vi "Coeficientes da norma - Uniforme.vi"(1 "Método de análise":T1(ring)=enum."Simplificado 2008", 2 "Tipo de roseta":u16(ring) items=["Roseta A", "Roseta B", "Roseta C"], 3 "Coluna":dbl=0.45 format="%#_13g", 4 "Linha":dbl=0.05 format="%#_13g") -> (0 "Coeficiente a e b":dbl[](array[numeric]))   [LabVIEW 2016]
uses:
  <vilib>/gmath/NI_Gmath.lvlib
panel:
  out "Linha":dbl[](array[numeric])
  out "Coluna":dbl[](array[numeric])
  out "Coeficiente B":dbl[][](array[numeric])
  out "Coeficiente A":dbl[][](array[numeric])
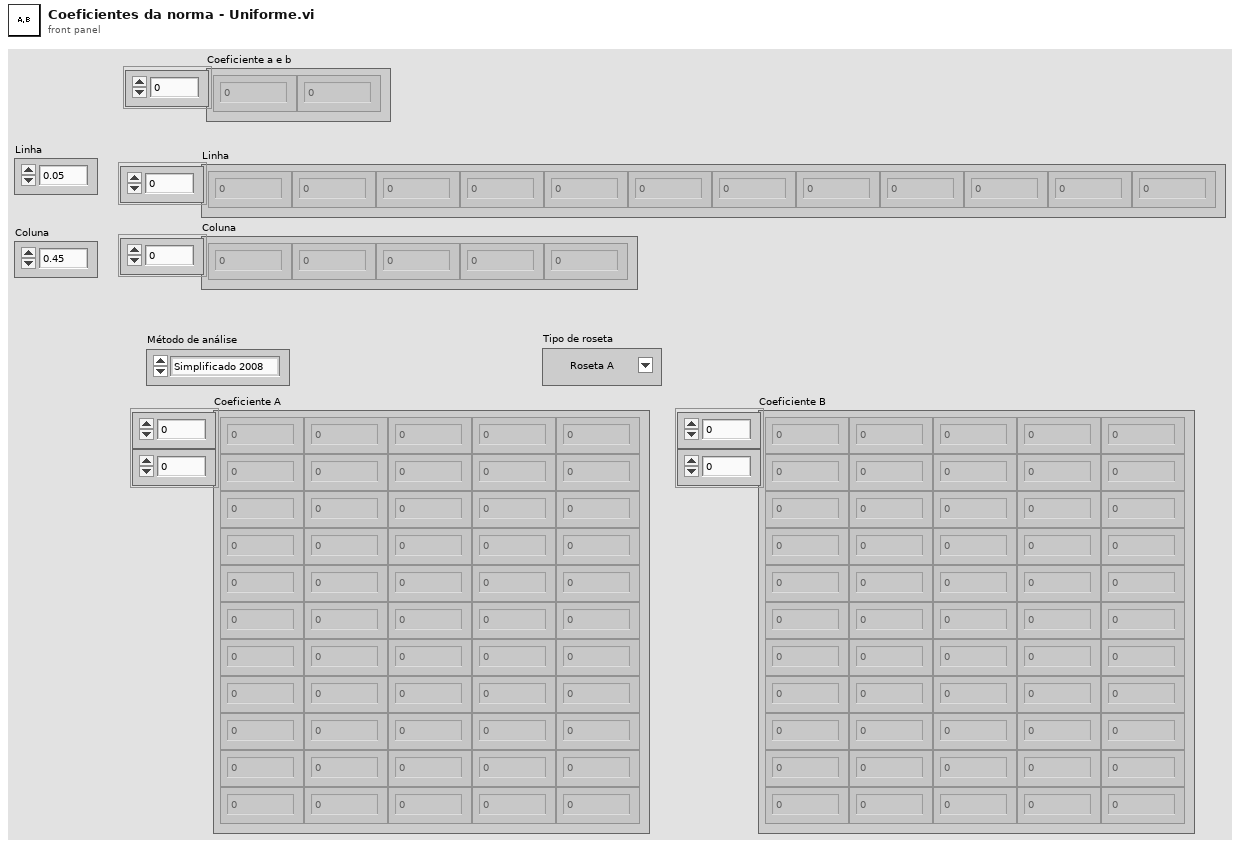
[diagram p1: front panel]
types:
  T1 = enum16{"Não uniforme 2013", "Simplificado 2013", "Simplificado 2008"}
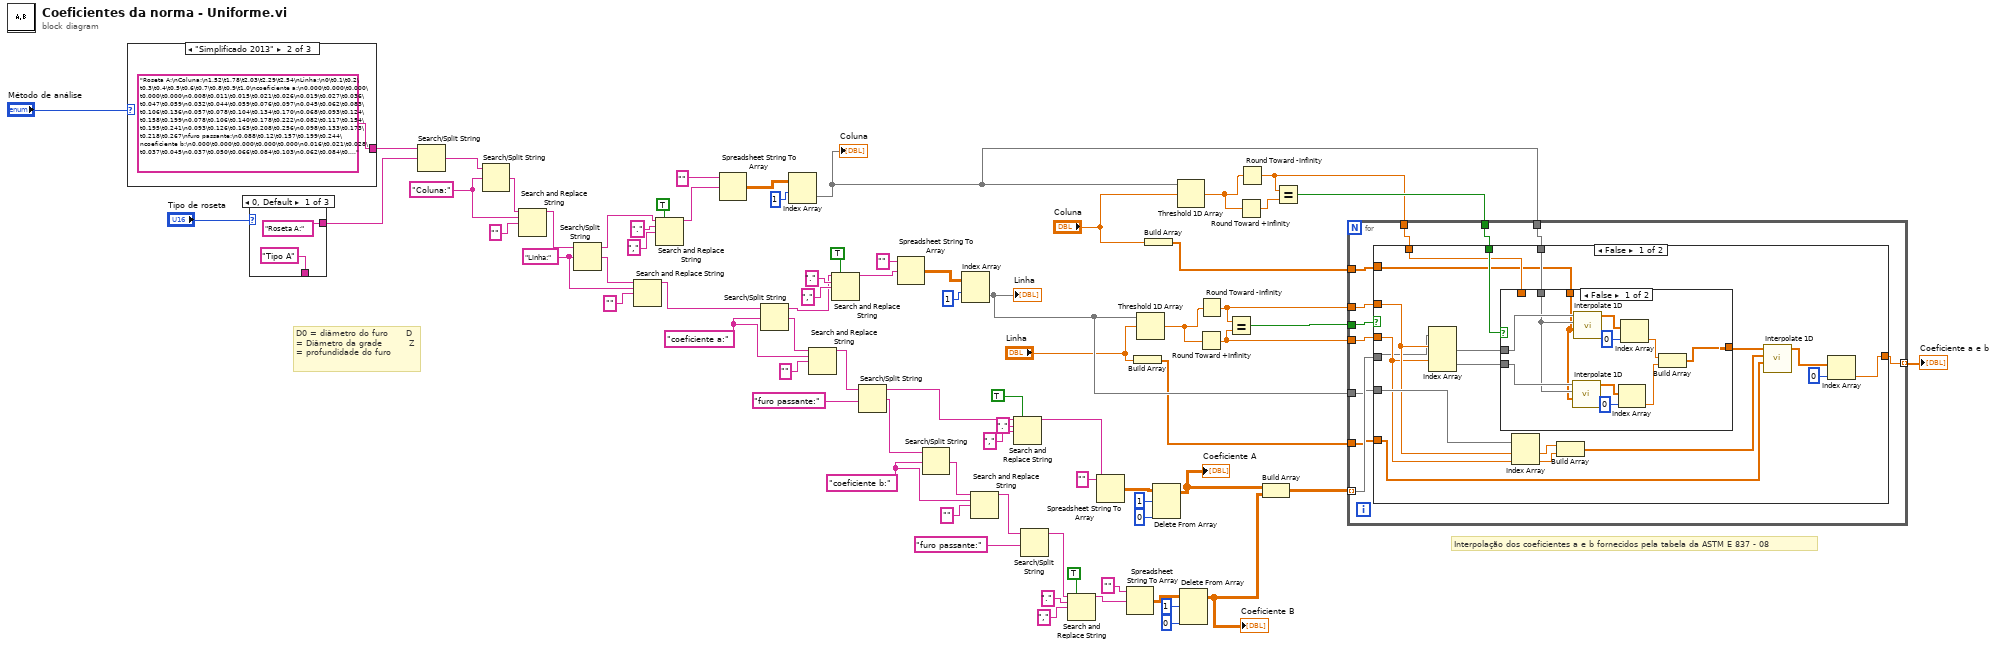
[diagram p0: block diagram]
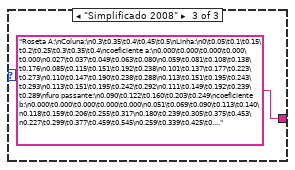
[diagram p3: hidden frame]
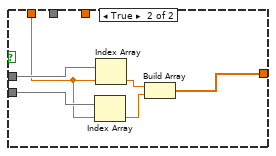
[diagram p4: hidden frame]
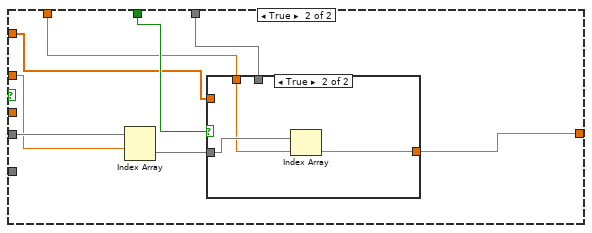
[diagram p5: hidden frame]
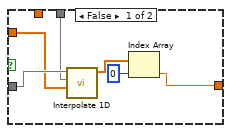
[diagram p6: hidden frame]
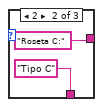
[diagram p7: hidden frame]
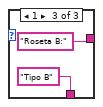
[diagram p8: hidden frame]
diagram:
  w40 = "Linha:" ("search string/char (-)")
  w42 = "Coluna:" ("search string/char (-)")
  w65 = "coeficiente b:"
  w74 = "coeficiente a:"
  # "Interpolação dos coeficientes a e b fornecidos pela tabela da ASTM E 837 - 08"
  # "D0 = diâmetro do furo      D = Diâmetro da grade         Z = profundidade do furo"
  n1 = case shown="\"Simplificado 2013\"" "Método de análise" {
    tunnel: [_ "Roseta A:\nColuna:\n1.52\t1.78\t2.03\t2.29\t2.54\nLinha:\n0\t0.1\t0.2\t0.3\t0.4\t0.5\t0.6\t0.7\t0.8\t0.9\t1.0\ncoeficiente a:\n0.000\t0.000\t0.000\t0.000\t0.000\n0.008\t0.011\t0.015\t0.021\t0.026\n0.019\t0.027\t0.036\t0.047\t0.059\n0.032\t0.044\t0.059\t0.076\t0.097\n0.045\t0.062\t0.083\t0.106\t0.136\n0.057\t0.078\t0.104\t0.134\t0.170\n0.068\t0.093\t0.124\t0.158\t0.199\n0.078\t0.106\t0.140\t0.178\t0.222\n0.082\t0.117\t0.154\t0.195\t0.241\n0.093\t0.126\t0.165\t0.208\t0.256\n0.098\t0.133\t0.173\t0.218\t0.267\nfuro passante:\n0.088\t0.12\t0.157\t0.199\t0.244\ncoeficiente b:\n0.000\t0.000\t0.000\t0.000\t0.000\n0.016\t0.021\t0.028\t0.037\t0.045\n0.037\t0.050\t0.066\t0.084\t0.103\n0.062\t0.084\t0.110\t0.137\t0.171\n0.088\t0.119\t0.155\t0.193\t0.241\n0.115\t0.154\t0.200\t0.248\t0.307\n0.140\t0.187\t0.242\t0.299\t0.367\n0.164\t0.218\t0.280\t0.345\t0.418\n0.185\t0.246\t0.314\t0.385\t0.463\n0.204\t0.270\t0.343\t0.419\t0.501\n0.221\t0.291\t0.370\t0.449\t0.533\nfuro passante:\n0.283\t0.371\t0.463\t0.554\t0.642\nCurvas limites:\ninferior:\n0\t0.1851\t0.4283\t0.6319\t0.7804\t0.8812\t0.9405\t0.9786\t1\nsuperior:\n0\t0.2559\t0.5602\t0.7845\t0.9198\t0.9874\t10.0143\t10.0143\t1 \n;\nRoseta B:\nColuna:\n1.52\t1.78\t2.03\t2.29\t2.54\nLinha:\n0\t0.1\t0.2\t0.3\t0.4\t0.5\t0.6\t0.7\t0.8\t0.9\t1.0\ncoeficiente a:\n0.000\t0.000\t0.000\t0.000\t0.000\n0.009\t0.012\t0.016\t0.022\t0.027\n0.021\t0.029\t0.039\t0.051\t0.063\n0.034\t0.047\t0.064\t0.082\t0.105\n0.048\t0.066\t0.089\t0.114\t0.146\n0.061\t0.084\t0.112\t0.143\t0.183\n0.073\t0.100\t0.132\t0.169\t0.213\n0.083\t0.114\t0.150\t0.190\t0.237\n0.092\t0.125\t0.164\t0.207\t0.256\n0.099\t0.134\t0.175\t0.221\t0.271\n0.105\t0.142\t0.184\t0.231\t0.282\nfuro passante:\n0.094\t0.128\t0.167\t0.212\t0.260\ncoeficiente b:\n0.000\t0.000\t0.000\t0.000\t0.000\n0.018\t0.024\t0.032\t0.041\t0.050\n0.042\t0.057\t0.074\t0.093\t0.115\n0.070\t0.094\t0.123\t0.153\t0.191\n0.100\t0.134\t0.175\t0.216\t0.270\n0.130\t0.174\t0.225\t0.278\t0.343\n0.159\t0.211\t0.272\t0.335\t0.409\n0.185\t0.246\t0.314\t0.385\t0.466\n0.209\t0.277\t0.352\t0.430\t0.515\n0.231\t0.305\t0.385\t0.468\t0.557\n0.249\t0.328\t0.413\t0.500\t0.592\nfuro passante:\n0.322\t0.421\t0.523\t0.621\t0.716\nCurvas limites:\ninferior:\n0\t0.1878\t0.4255\t0.6349\t0.7818\t0.8809\t0.9430\t0.9785\t1\nsuperior:\n0\t0.2623\t0.5695\t0.7966\t0.9297\t0.9964\t10.0143\t10.0136\t1\n;\nRoseta C:\nColuna:\n1.52\t1.78\t2.03\t2.29\t2.54\nLinha:\n0\t0.1\t0.2\t0.3\t0.4\t0.5\t0.6\t0.7\t0.8\t0.9\t1.0\ncoeficiente a:\n0.000\t0.000\t0.000\t0.000\t0.000\n0.019\t0.027\t0.038\t0.050\t0.061\n0.046\t0.064\t0.086\t0.111\t0.139\n0.076\t0.105\t0.141\t0.182\t0.235\n0.106\t0.147\t0.197\t0.253\t0.324\n0.134\t0.186\t0.248\t0.316\t0.400\n0.160\t0.221\t0.292\t0.371\t0.464\n0.182\t0.250\t0.330\t0.416\t0.515\n0.201\t0.275\t0.361\t0.453\t0.556\n0.217\t0.296\t0.386\t0.482\t0.588\n0.230\t0.312\t0.405\t0.505\t0.613\nfuro passante:\n0.246\t0.335\t0.437\t0.553\t0.681\ncoeficiente b:\n0.000\t0.000\t0.000\t0.000\t0.000\n0.032\t0.043\t0.056\t0.070\t0.082\n0.076\t0.103\t0.132\t0.161\t0.193\n0.128\t0.172\t0.221\t0.269\t0.333\n0.184\t0.246\t0.315\t0.383\t0.468\n0.240\t0.320\t0.407\t0.490\t0.589\n0.293\t0.389\t0.491\t0.587\t0.695\n0.343\t0.452\t0.566\t0.673\t0.784\n0.387\t0.507\t0.631\t0.745\t0.858\n0.427\t0.556\t0.687\t0.806\t0.918\n0.461\t0.597\t0.734\t0.856\t0.968\nfuro passante:\n0.519\t0.648\t0.758\t0.831\t0.860\nCurvas limites:\ninferior:\n0\t0.1632\t0.3793\t0.5860\t0.7365\t0.8482\t0.9213\t0.9680\t1\nsuperior:\n0\t0.2079\t0.4643\t0.6754\t0.8238\t0.9099\t0.9608\t0.9844\t1\n;" ("text") "Roseta A:\nColuna:\n0.3\t0.35\t0.4\t0.45\t0.5\nLinha:\n0\t0.05\t0.1\t0.15\t0.2\t0.25\t0.3\t0.35\t0.4\ncoeficiente a:\n0.000\t0.000\t0.000\t0.000\t0.000\n0.027\t0.037\t0.049\t0.063\t0.080\n0.059\t0.081\t0.108\t0.138\t0.176\n0.085\t0.115\t0.151\t0.192\t0.238\n0.101\t0.137\t0.177\t0.223\t0.273\n0.110\t0.147\t0.190\t0.238\t0.288\n0.113\t0.151\t0.195\t0.243\t0.293\n0.113\t0.151\t0.195\t0.242\t0.292\n0.111\t0.149\t0.192\t0.239\t0.289\nfuro passante:\n0.090\t0.122\t0.160\t0.203\t0.249\ncoeficiente b:\n0.000\t0.000\t0.000\t0.000\t0.000\n0.051\t0.069\t0.090\t0.113\t0.140\n0.118\t0.159\t0.206\t0.255\t0.317\n0.180\t0.239\t0.305\t0.375\t0.453\n0.227\t0.299\t0.377\t0.459\t0.545\n0.259\t0.339\t0.425\t0.513\t0.603\n0.279\t0.364\t0.454\t0.546\t0.638\n0.292\t0.379\t0.472\t0.566\t0.657\n0.297\t0.387\t0.482\t0.576\t0.668\nfuro passante:\n0.288\t0.377\t0.470\t0.562\t0.651\nCurvas limites:\ninferior:\n0\t0.1851\t0.4283\t0.6319\t0.7804\t0.8812\t0.9405\t0.9786\t1\nsuperior:\n0\t0.2559\t0.5602\t0.7845\t0.9198\t0.9874\t10.0143\t10.0143\t1 \n;\nRoseta B:\nColuna:\n0.3\t0.35\t0.4\t0.45\t0.5\nLinha:\n0\t0.05\t0.1\t0.15\t0.2\t0.25\t0.3\t0.35\t0.4\ncoeficiente a:\n0.000\t0.000\t0.000\t0.000\t0.000\n0.029\t0.039\t0.053\t0.068\t0.086\n0.063\t0.087\t0.116\t0.148\t0.189\n0.090\t0.123\t0.162\t0.205\t0.254\n0.107\t0.145\t0.189\t0.236\t0.289\n0.116\t0.156\t0.202\t0.251\t0.305\n0.120\t0.160\t0.206\t0.256\t0.309\n0.120\t0.160\t0.206\t0.256\t0.308\n0.118\t0.158\t0.203\t0.253\t0.305\nfuro passante:\n0.096\t0.131\t0.171\t0.216\t0.265\ncoeficiente b:\n0.000\t0.000\t0.000\t0.000\t0.000\n0.058\t0.078\t0.102\t0.127\t0.157\n0.134\t0.179\t0.231\t0.286\t0.355\n0.203\t0.269\t0.343\t0.419\t0.504\n0.256\t0.336\t0.423\t0.511\t0.605\n0.292\t0.381\t0.476\t0.571\t0.668\n0.315\t0.410\t0.509\t0.609\t0.707\n0.330\t0.427\t0.529\t0.631\t0.730\n0.337\t0.437\t0.541\t0.644\t0.743\nfuro passante:\n0.329\t0.428\t0.531\t0.630\t0.725\nCurvas limites:\ninferior:\n0\t0.1878\t0.4255\t0.6349\t0.7818\t0.8809\t0.9430\t0.9785\t1\nsuperior:\n0\t0.2623\t0.5695\t0.7966\t0.9297\t0.9964\t10.0143\t10.0136\t1\n;\nRoseta C:\nColuna:\n0.4\t0.45\t0.5\t0.55\t0.6\nLinha:\n0\t0.05\t0.1\t0.15\t0.2\t0.25\t0.3\t0.35\t0.4\ncoeficiente a:\n0.000\t0.000\t0.000\t0.000\t0.000\n0.065\t0.084\t0.106\t0.130\t0.157\n0.147\t0.191\t0.238\t0.293\t0.361\n0.218\t0.281\t0.347\t0.420\t0.506\n0.270\t0.343\t0.421\t0.504\t0.595\n0.302\t0.381\t0.465\t0.554\t0.648\n0.321\t0.403\t0.491\t0.583\t0.679\n0.331\t0.415\t0.505\t0.599\t0.698\n0.336\t0.421\t0.512\t0.608\t0.709\nfuro passante:\n0.316\t0.399\t0.494\t0.597\t0.707\ncoeficiente b:\n0.000\t0.000\t0.000\t0.000\t0.000\n0.105\t0.132\t0.158\t0.185\t0.217\n0.250\t0.314\t0.373\t0.440\t0.519\n0.391\t0.484\t0.570\t0.658\t0.754\n0.506\t0.617\t0.719\t0.816\t0.912\n0.591\t0.712\t0.823\t0.923\t10.015\n0.650\t0.778\t0.893\t0.994\t10.081\n0.690\t0.822\t0.939\t10.041\t10.125\n0.719\t0.851\t0.970\t10.073\t10.154\nfuro passante:\n0.623\t0.723\t0.799\t0.847\t0.859\nCurvas limites:\ninferior:\n0\t0.1632\t0.3793\t0.5860\t0.7365\t0.8482\t0.9213\t0.9680\t1\nsuperior:\n0\t0.2079\t0.4643\t0.6754\t0.8238\t0.9099\t0.9608\t0.9844\t1\n;" ("text")] -> w2
    frame "Não uniforme 2013", Default {
    }
    frame "Simplificado 2013" {
    }
    frame "Simplificado 2008" {
    }
  }
  n2 = case shown="0, Default" "Tipo de roseta" {
    tunnel: ["Roseta A:" "Roseta C:" "Roseta B:"] -> w75
    tunnel: ["Tipo A" "Tipo C" "Tipo B"] -> _
    frame 0, Default {
    }
    frame 2 {
    }
    frame 1 {
    }
  }
  n3 = Search/Split String(string=w2, search string/char (-)=w75) -> (match + rest of string=w45:string)  [unwired: 1 in, 2 out]
  n4 = Search/Split String(string=w45, search string/char (-)=w42) -> (match + rest of string=w43:string)  [unwired: 1 in, 2 out]
  n5 = Search and Replace String(input string=w43, search string=w42, replace string="" ("replace string (\"\")")) -> (result string=w38:string)  [unwired: 5 in, 3 out]
  n6 = Search/Split String(string=w38, search string/char (-)=w40) -> (substring before match=w31:string, match + rest of string=w37:string)  [unwired: 1 in, 1 out]
  n7 = Search and Replace String(input string=w37, search string=w40, replace string="" ("replace string (\"\")")) -> (result string=w39:string)  [unwired: 5 in, 3 out]
  n8 = Search and Replace String(replace all?=TRUE ("replace all? (F)"), input string=w31, search string=".", replace string="," ("replace string (\"\")")) -> (result string=w30:string)  [unwired: 4 in, 3 out]
  n9 = Spreadsheet String To Array(format string="", spreadsheet string=w30) -> (array=w24:dbl[][])  [unwired: 2 in]
  n10 = Search/Split String(string=w39, search string/char (-)=w74) -> (substring before match=w26:string, match + rest of string=w70:string)  [unwired: 1 in, 1 out]
  n11 = Index Array(array=w24, index (row)=1 ("disabled index (col)")) -> (element=w13:dbl[])  [unwired: 1 in]
  "Coluna" <- w13
  n12 = Search and Replace String(input string=w70, search string=w74, replace string="" ("replace string (\"\")")) -> (result string=w72:string)  [unwired: 5 in, 3 out]
  n13 = Search and Replace String(replace all?=TRUE ("replace all? (F)"), input string=w26, search string=".", replace string="," ("replace string (\"\")")) -> (result string=w25:string)  [unwired: 4 in, 3 out]
  n14 = Search/Split String(string=w72, search string/char (-)="furo passante:") -> (substring before match=w62:string, match + rest of string=w64:string)  [unwired: 1 in, 1 out]
  n15 = Spreadsheet String To Array(format string="", spreadsheet string=w25) -> (array=w23:dbl[][])  [unwired: 2 in]
  n16 = Search/Split String(string=w64, search string/char (-)=w65) -> (match + rest of string=w69:string)  [unwired: 1 in, 2 out]
  n17 = Index Array(array=w23, index (row)=1 ("disabled index (col)")) -> (element=w9:dbl[])  [unwired: 1 in]
  "Linha" <- w9
  n18 = Search and Replace String(input string=w69, search string=w65, replace string="" ("replace string (\"\")")) -> (result string=w67:string)  [unwired: 5 in, 3 out]
  n19 = Search and Replace String(replace all?=TRUE ("replace all? (F)"), input string=w62, search string=".", replace string="," ("replace string (\"\")")) -> (result string=w55:string)  [unwired: 4 in, 3 out]
  n20 = Search/Split String(string=w67, search string/char (-)="furo passante:") -> (substring before match=w58:string)  [unwired: 1 in, 2 out]
  n21 = Search and Replace String(replace all?=TRUE ("replace all? (F)"), input string=w58, search string=".", replace string="," ("replace string (\"\")")) -> (result string=w54:string)  [unwired: 4 in, 3 out]
  n22 = Spreadsheet String To Array(format string="", spreadsheet string=w55) -> (array=w46:dbl[][])  [unwired: 2 in]
  n23 = Spreadsheet String To Array(format string="", spreadsheet string=w54) -> (array=w51:dbl[][])  [unwired: 2 in]
  n24 = Build Array("Linha") -> (w7:dbl[])
  n25 = Threshold 1D Array(2:"Linha", 3:w9) -> (0:w20:dbl)  [unwired: 1 in]
  n26 = Build Array("Coluna") -> (w11:dbl[])
  n27 = Delete From Array(array=w46, length=1, index (row)=0) -> (array with subset deleted=w3:dbl[][])  [unwired: 1 in, 1 out]
  "Coeficiente A" <- w3
  n28 = Threshold 1D Array(2:"Coluna", 3:w13) -> (0:w17:dbl)  [unwired: 1 in]
  n29 = Delete From Array(array=w51, length=1, index (row)=0) -> (array with subset deleted=w6:dbl[][])  [unwired: 1 in, 1 out]
  "Coeficiente B" <- w6
  n30 = Round Toward +Infinity(x=w20) -> (ceil(x): smallest int >= x=w10:dbl)
  n31 = Round Toward -Infinity(1:w20) -> (0:w18:dbl)
  n32 = Equal?(x=w18, y=w10) -> (x = y?=w19:bool)
  n33 = Round Toward +Infinity(x=w17) -> (ceil(x): smallest int >= x=w16:dbl)
  n34 = Round Toward -Infinity(1:w17) -> (0:w14:dbl)
  n35 = Build Array(w3, w6) -> (w5:dbl[][][])
  n36 = Equal?(x=w14, y=w16) -> (x = y?=w15:bool)
  n37 = for {
    tunnel: w19 -> [w95]
    tunnel: w18 -> [w94]
    tunnel: w15 -> [w93]
    tunnel: w14 -> [w92]
    tunnel: [w91] -> w4 mode=indexing
    tunnel: w13 -> [w90]
    tunnel: w11 -> [w89]
    tunnel: w5 -> [w88] mode=indexing
    tunnel: w10 -> [w87]
    tunnel: w9 -> [w86]
    tunnel: w7 -> [w85]
    n38 = case shown="False" w95 {
      tunnel: w94 -> [w107 w137]
      tunnel: w88 -> [w96 w138]
      tunnel: w93 -> [w113 w136]
      tunnel: w92 -> [w110 w134]
      tunnel: [w99 w133] -> w91
      tunnel: w90 -> [w98 w132]
      tunnel: w89 -> [w97 w131]
      tunnel: w87 -> [w106 _]
      tunnel: w86 -> [w108 _]
      tunnel: w85 -> [w102 _]
      frame False {
        n39 = Index Array(array=w96, index (row) #1=w107, index (row) #2=w106) -> (element #1=w112:dbl[], element #2=w111:dbl[])  [unwired: 2 in]
        n40 = case shown="False" w113 {
          tunnel: w112 -> [w124 w130]
          tunnel: w111 -> [w123 w129]
          tunnel: w110 -> [_ w128]
          tunnel: [w114 w125] -> w109
          tunnel: w98 -> [w122 _]
          tunnel: w97 -> [w121 _]
          frame False {
            n41 = call <vilib>:"Interpolate 1D.vi"("xi"=w121, "X"=w122, "Y"=w123) -> ("yi"=w117:dbl[])  [unwired: 6 in, 2 out]
            n42 = call <vilib>:"Interpolate 1D.vi"("xi"=w121, "X"=w122, "Y"=w124) -> ("yi"=w119:dbl[])  [unwired: 6 in, 2 out]
            n43 = Index Array(array=w117, index=0) -> (element=w115:dbl)
            n44 = Index Array(array=w119, index=0) -> (element=w116:dbl)
            n45 = Build Array(w116, w115) -> (w114:dbl[])
          }
          frame True {
            n46 = Index Array(array=w129, index=w128) -> (element=w126:dbl)
            n47 = Index Array(array=w130, index=w128) -> (element=w127:dbl)
            n48 = Build Array(w127, w126) -> (w125:dbl[])
          }
        }
        n49 = Index Array(array=w108, index #1=w107, index #2=w106) -> (element #1=w105:dbl, element #2=w104:dbl)
        n50 = Build Array(w105, w104) -> (w103:dbl[])
        n51 = call <vilib>:"Interpolate 1D.vi"("xi"=w102, "X"=w103, "Y"=w109) -> ("yi"=w101:dbl[])  [unwired: 6 in, 2 out]
        n52 = Index Array(array=w101, index=0) -> (element=w99:dbl)
      }
      frame True {
        n53 = Index Array(array=w138, index (row)=w137) -> (element=w135:dbl[])  [unwired: 1 in]
        n54 = case shown="True" w136 {
          tunnel: w135 -> [w144 w147]
          tunnel: w134 -> [_ w146]
          tunnel: [w139 w145] -> w133
          tunnel: w132 -> [w143 _]
          tunnel: w131 -> [w142 _]
          frame False {
            n55 = call <vilib>:"Interpolate 1D.vi"("xi"=w142, "X"=w143, "Y"=w144) -> ("yi"=w141:dbl[])  [unwired: 6 in, 2 out]
            n56 = Index Array(array=w141, index=0) -> (element=w139:dbl)
          }
          frame True {
            n57 = Index Array(array=w147, index=w146) -> (element=w145:dbl)
          }
        }
      }
    }
  }
  "Coeficiente a e b" <- w4
